vi "Nonlinear Model.vi"(1 "State variables, x":dbl[](array[numeric]) format="%.3f", 2 "Contro yaw, f":dbl=1.0 min=-40.0 max=40.0 step=5.0 format="%.2f", 3 "Control pitch, q":dbl=1.0 min=-40.0 max=40.0 step=5.0 format="%.2f") -> (0 "New state variables":dbl[](array[numeric]) format="%.3f")   [LabVIEW 2022 SP3]
uses:
  <vilib>/imath/engines/lvmath2/RunTimeEngine/IndexRead/NIMS V(S).vi
  <instcachedir>/0/NIMS V(S)_0488751826AF41519A22953C041130DC.lvgen/NIMS V(S)_0488751826AF41519A22953C041130DC_000.vi
  <vilib>/imathl/engines/lvmath/Functions/Error Handling/Create Error.vi
  <vilib>/imath/engines/lvmath2/RunTimeEngine/ErrorHandling/NIMS_Create Error From Enums.vi
  <vilib>/imath/engines/lvmath2/RunTimeEngine/ArithmeticOperatorToken/NIMS_ArithmeticOperator_multmx(M,CV)-internal.vi
  <instcachedir>/0/NIMS_ArithmeticOperator_multmx(M,CV)-internal_4CF26FF1FDF34EBEB91D740490649658.lvgen/NIMS_ArithmeticOperator_multmx(M,CV)-internal_4CF26FF1FDF34EBEB91D740490649658_001.vi
  <vilib>/imath/engines/lvmath2/RunTimeEngine/ArithmeticOperatorToken/NIMS_ArithmeticOperator_plus.vi
  <instcachedir>/0/NIMS_ArithmeticOperator_plus_3E2F46F6B6A2434E909AF418D4802C21.lvgen/NIMS_ArithmeticOperator_plus_3E2F46F6B6A2434E909AF418D4802C21_004.vi
  <vilib>/imath/engines/lvmath2/RunTimeEngine/NodeEndStatement/NIMS_NodeEndStatement_Output.vi
  <instcachedir>/0/NIMS_NodeEndStatement_Output_53EC0D466D134D7ABD903AC30B43404B.lvgen/NIMS_NodeEndStatement_Output_53EC0D466D134D7ABD903AC30B43404B_005.vi
  <vilib>/imath/engines/lvmath2/RunTimeEngine/ErrorHandling/NIMS_Finalize Error.vi
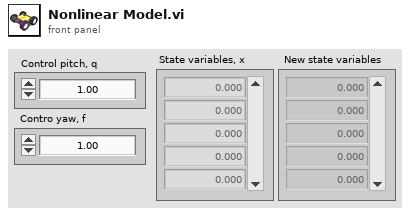
[diagram p1: front panel]
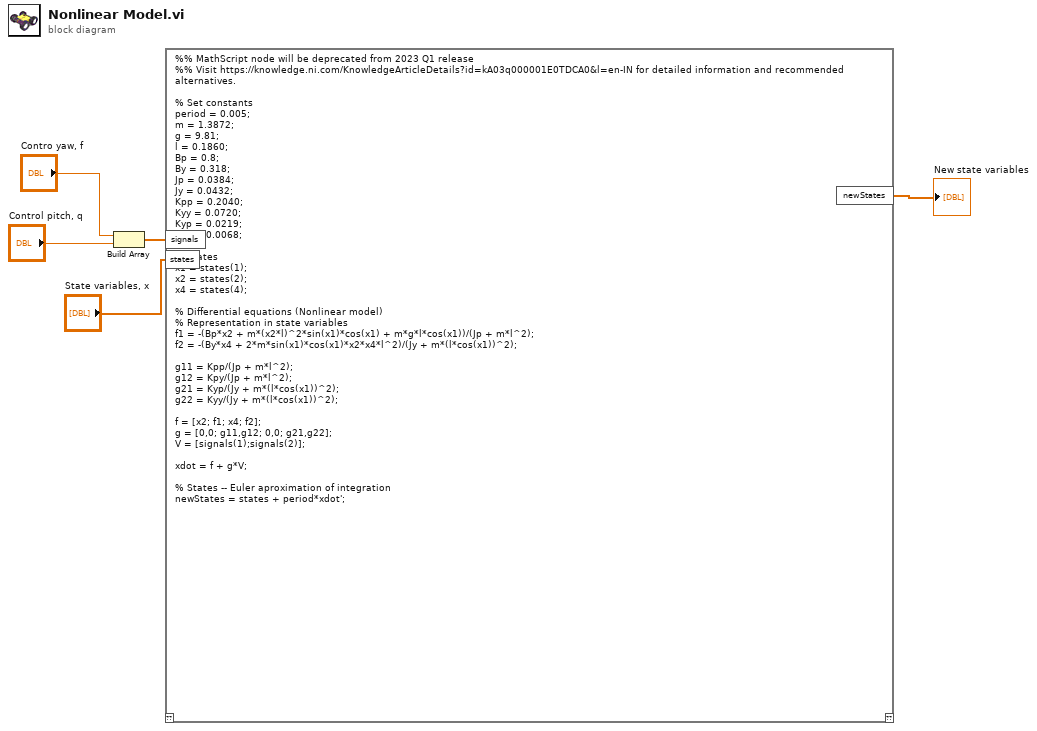
[diagram p0: block diagram]
diagram:
  n1 = Build Array("Contro yaw, f", "Control pitch, q") -> (w3:dbl[])
  n2 = mathscript code="%% MathScript node will be deprecated from 2023 Q1 release\n%% Visit https://knowledge.ni.com/KnowledgeArticleDetails?id=kA03q000001E0TDCA0&l=en-IN for detailed information and recommended alternatives.\n\n% Set constants\nperiod = 0.005;\nm = 1.3872;\ng = 9.81;\nl = 0.1860;\nBp = 0.8;\nBy = 0.318;\nJp = 0.0384;\nJy = 0.0432;\nKpp = 0.2040;\nKyy = 0.0720;\nKyp = 0.0219;\nKpy = 0.0068;\n\n% States\nx1 = states(1);\nx2 = states(2);\nx4 = states(4);\n\n% Differential equations (Nonlinear model)\n% Representation in state variables\nf1 = -(Bp*x2 + m*(x2*l)^2*sin(x1)*cos(x1) + m*g*l*cos(x1))/(Jp + m*l^2);\nf2 = -(By*x4 + 2*m*sin(x1)*cos(x1)*x2*x4*l^2)/(Jy + m*(l*cos(x1))^2);\n        \ng11 = Kpp/(Jp + m*l^2);\ng12 = Kpy/(Jp + m*l^2);\ng21 = Kyp/(Jy + m*(l*cos(x1))^2);\ng22 = Kyy/(Jy + m*(l*cos(x1))^2);\n        \nf = [x2; f1; x4; f2];\ng = [0,0; g11,g12; 0,0; g21,g22];\nV = [signals(1);signals(2)];\n        \nxdot = f + g*V;\n\n% States -- Euler aproximation of integration\nnewStates = states + period*xdot';"("signals"=w3, "states"="State variables, x") -> ("newStates"=→"New state variables":dbl[])  [unwired: 1 in, 1 out]
